vi "DHE_get_intdelay.vi"(0 "fd in":i32, 11 "error in (no error)":errorcluster) -> (4 "fd out":i32, 6 "msdelay":sgl, 15 "error out":errorcluster)   [LabVIEW 2016]
doc: "This VI closes the I/O interface with the instrument."
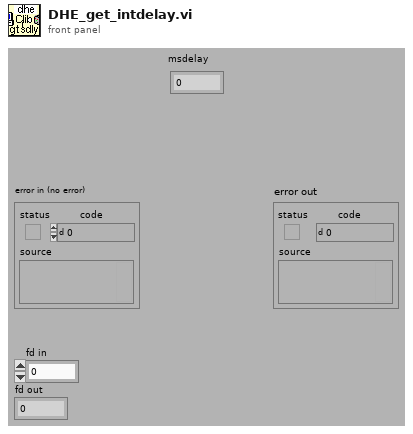
[diagram p1: front panel]
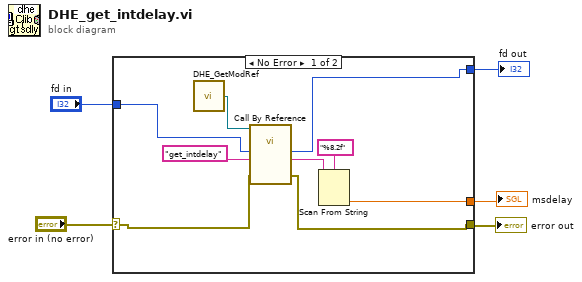
[diagram p0: block diagram]
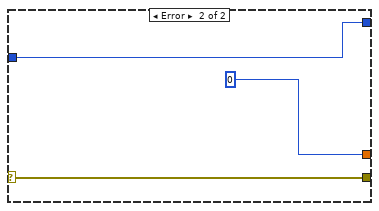
[diagram p2: hidden frame]
diagram:
  n1 = case shown="No Error" "error in (no error)" {
    selector: "error in (no error)" -> [w7 w17]
    tunnel: [w6 w17] -> w5
    tunnel: [w8 0 ("sequence")] -> w1
    tunnel: "fd in" -> [w10 w15]
    tunnel: [w9 w15] -> w2
    frame No Error {
      n2 = call "DHE_GetModRef.vi"() -> ("DHE_ModRef"=w14:refnum<vi>)  [unwired: 9 out]
      n3 = call-by-ref "?"(reference=w14, "error in (no error)"=w7, "function"="get_intdelay", "fd in"=w10) -> ("error out"=w6:errorcluster, "str result"=w12:string, "fd out"=w9:i32)  [unwired: 6 in, 3 out]
      n4 = Scan From String(format string="%8.2f", input string=w12) -> (output 1=w8:dbl)  [unwired: 2 in, 4 out]
    }
    frame Error {
    }
  }
  "error out" <- w5
  "msdelay" <- w1
  "fd out" <- w2
